vi "optionsAcq_channel_offset.vi"(8 "error in (no error)":errorcluster, 9 "readWrite":enum16{"read", "write"}(ring), 10 "detector offset":u16, 11 "OSAchannel in":refnum<class "OSAchannel.lvclass">) -> (0 "error out":errorcluster, 1 "status ftsLib":i32, 2 "offset read":i32, 3 "OSAchannel out":refnum<class "OSAchannel.lvclass">)   [LabVIEW 2010, in "OSAchannel.lvclass"]
uses:
  OSAchannel.lvclass
  OSAchannel.lvclass/OSAchannel.ctl
  OSA20X_misc.lvlib
  FTSLib.dll
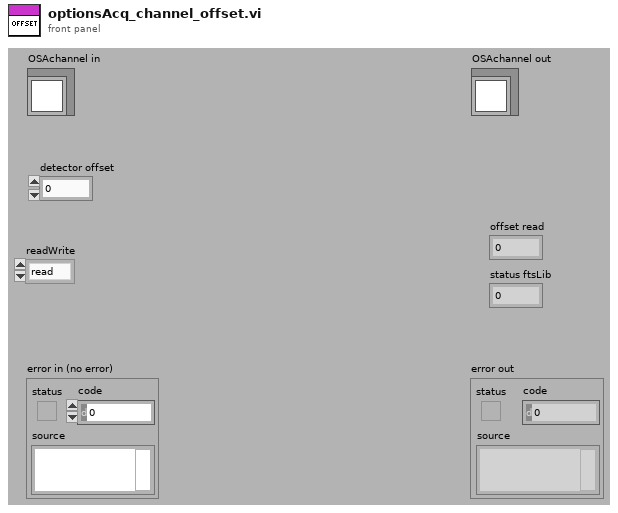
[diagram p1: front panel]
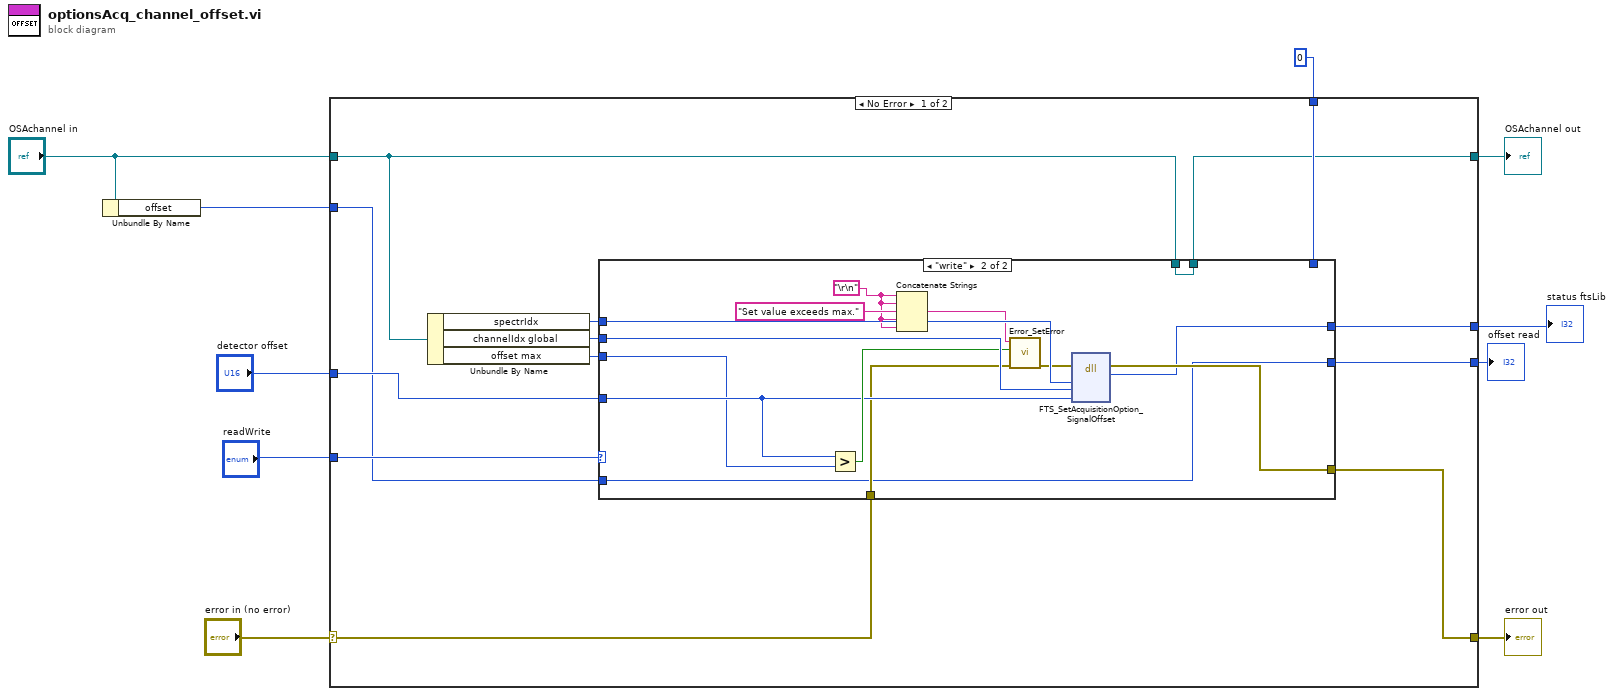
[diagram p0: block diagram]
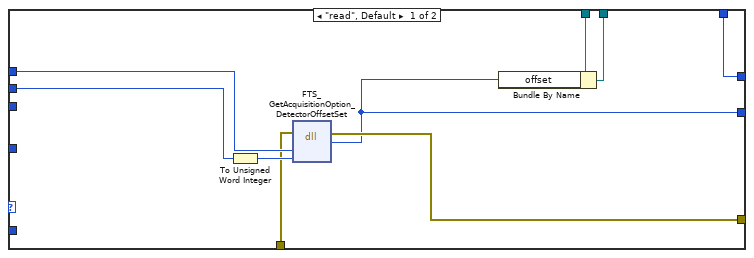
[diagram p2: hidden frame]
diagram:
  n1 = Unbundle By Name("OSAchannel in") -> ("offset"=w2:i32)
  n2 = case shown="No Error" "error in (no error)" {
    selector: "error in (no error)" -> [w19 w50]
    tunnel: [w16 w50] -> w9
    tunnel: [w14 w49] -> w8
    tunnel: "OSAchannel in" -> [w15 w49]
    tunnel: "readWrite" -> [w20 _]
    tunnel: "detector offset" -> [w18 _]
    tunnel: 0 ("status") -> [w17 w48]
    tunnel: [w13 w48] -> w4
    tunnel: w2 -> [w12 w47]
    tunnel: [w11 w47] -> w1
    frame No Error {
      n3 = Unbundle By Name(w15) -> ("spectrIdx"=w23:u16, "channelIdx global"=w22:u16, "offset max"=w21:u16)
      n4 = case shown="\"write\"" w20 {
        tunnel: w23 -> [w32 w46]
        tunnel: w22 -> [w31 w45]
        tunnel: [w24 w33] -> w11
        tunnel: [w29 w44] -> w16
        tunnel: w15 -> [w28 w43]
        tunnel: [w27 w43] -> w14
        tunnel: w17 -> [w25 _]
        tunnel: w19 -> [w26 w35]
        tunnel: [w25 w34] -> w13
        tunnel: w21 -> [_ w36]
        tunnel: w18 -> [_ w37]
        tunnel: w12 -> [_ w33]
        frame "read", Default {
          n5 = To Unsigned Word Integer(number=w31) -> (unsigned 16bit integer=w30:u16)
          n6 = dll-call lib="FTSLib.dll" fn="FTS_GetAcquisitionOption_DetectorOffsetSet"(error in=w26, "spectrIdx"=w32, "channeldx"=w30) -> (error out=w29:errorcluster, "offset"=w24:i32)  [unwired: 4 in, 1 out]
          n7 = Bundle By Name(cluster=w28, "offset"=w24) -> (w27:refnum<class "OSAchannel.lvclass">)
        }
        frame "write" {
          w38 = "\r\n"
          n8 = Greater?(x=w37, y=w36) -> (0:w39:bool)
          n9 = Concatenate Strings(w38, w38, "Set value exceeds max." ("source(\"\")"), w38, w38) -> (w40:string)
          n10 = call "Error_SetError.vi"("error in"=w35, "status (true)"=w39, "source(\"\")"=w40) -> ("error out"=w42:errorcluster)  [unwired: 4 in]
          n11 = dll-call lib="FTSLib.dll" fn="FTS_SetAcquisitionOption_SignalOffset"(error in=w42, "spectrIdx"=w46, "channeldx"=w45, "offset"=w37) -> (error out=w44:errorcluster, "status"=w34:i32)  [unwired: 5 in, 1 out]
        }
      }
    }
    frame Error {
    }
  }
  "error out" <- w9
  "OSAchannel out" <- w8
  "status ftsLib" <- w4
  "offset read" <- w1
